vi "API_POST.vi"(8 "error in (no error)":errorcluster, 9 "buffer":string, 10 "endpoint":string, 11 "DB_API.lvclass":refnum<class "DB_API.lvclass">) -> (0 "error out":errorcluster, 2 "body":string, 3 "output cluster":refnum<class "DB_API.lvclass">)   [LabVIEW 2024, in "DB_API.lvclass"]
uses:
  DB_API.lvclass
  DB_API.lvclass/DB_API.ctl
  <vilib>/httpClient/POSTBuffer.vi
  <vilib>/httpClient/LabVIEWHTTPClient.lvlib
panel:
  out "error out 2":errorcluster
  out "concatenated string":string
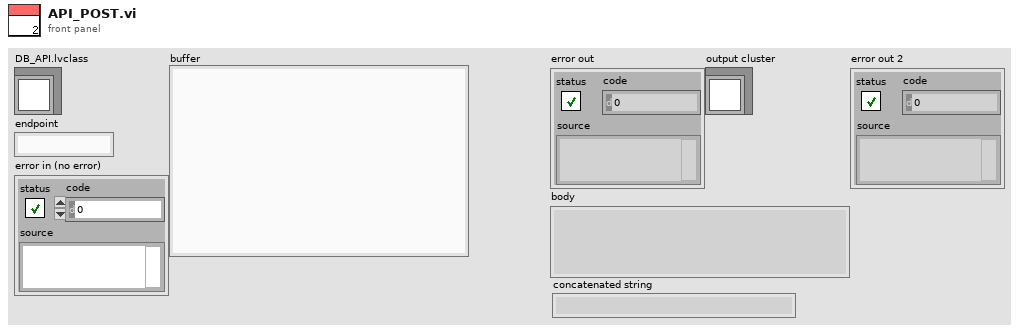
[diagram p1: front panel]
types:
  T1 = typedef "LabVIEWHTTPClient.lvlib/ClientHandle.ctl" = refnum<k1>
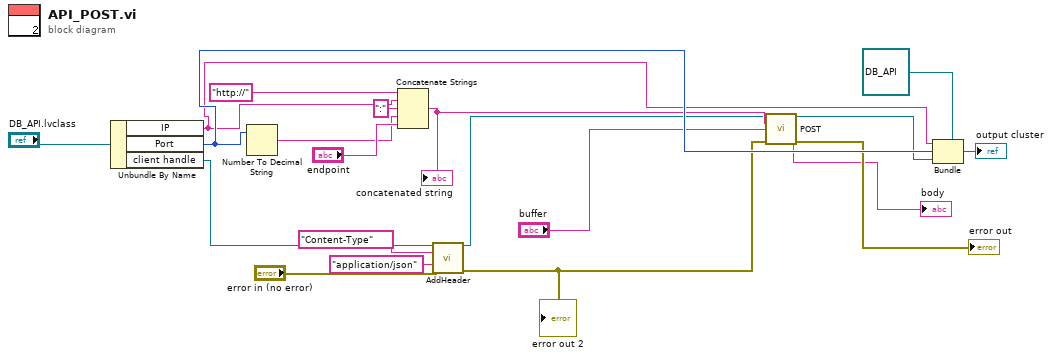
[diagram p0: block diagram]
diagram:
  n1 = Unbundle By Name("DB_API.lvclass") -> ("IP"=w16:string, "Port"=w17:u32, "client handle"=w6:T1)
  n2 = Number To Decimal String(number=w17) -> (decimal integer string=w13:string)  [unwired: 1 in]
  n3 = Concatenate Strings("http://" ("string"), w16, ":" ("string"), w13, "endpoint") -> (w12:string)
  "concatenated string" <- w12
  n4 = call <vilib>:"AddHeader.vi"("client handle"=w6, "header"="Content-Type", "value"="application/json", "error in (no error)"="error in (no error)") -> ("client handle out"=w2:T1, "error out"=w1:errorcluster)  [unwired: 10 in]
  "error out 2" <- w1
  n5 = call-poly <vilib>:"POST.vi"("client handle"=w2, "url"=w12, "buffer"="buffer", "error in (no error)"=w1) -> ("client handle out"=w9:T1, "body"=→"body":string, "error out"=→"error out":errorcluster)  [unwired: 8 in, 1 out]
  n6 = Bundle(cluster=refnum<class "DB_API.lvclass"> refnum ("DB_API.lvclass"), w16, w17, w9) -> (→"output cluster":refnum<class "DB_API.lvclass">)
